vi "Read Source.vi"(8 "Error In":errorcluster, 11 "Node In":refnum<class "NonTerminal.lvclass">) -> (0 "Error Out":errorcluster, 2 "Source":string, 3 "Node Out":refnum<class "NonTerminal.lvclass">)   [LabVIEW 2018, in "Toolkit.lvlib" / "Nodes.lvlib" / "NonTerminal.lvclass"]
uses:
  NonTerminal.lvclass
  Abstract/Abstract.lvclass
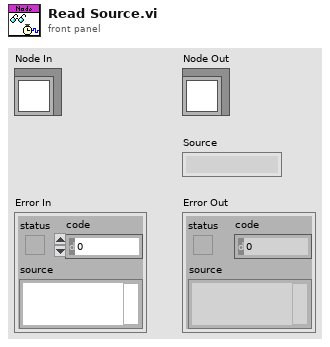
[diagram p1: front panel]
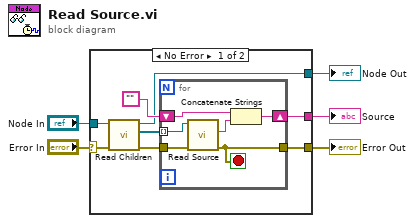
[diagram p0: block diagram]
diagram:
  n1 = case shown="No Error" "Error In" {
    selector: "Error In" -> [w10 w20]
    tunnel: "Node In" -> [w9 w21]
    tunnel: [w8 w21] -> w3
    tunnel: [w7 _] -> w2
    tunnel: [w6 w20] -> w1
    frame No Error {
      n2 = call-dynamic "Read Children.vi"("Error In"=w10, "Non-Terminal In"=w9) -> ("Error Out"=w11:errorcluster, "Children"=w12:refnum<class "Abstract.lvclass">[], "Non-Terminal Out"=w8:refnum<class "NonTerminal.lvclass">)  [unwired: 7 in]
      n3 = for {
        shift-right: [w18] -> w7
        shift-left: "" -> [w19]
        tunnel: w12 -> [w16] mode=indexing
        tunnel: w11 -> [w15]
        tunnel: [w14] -> w6
        stop <- w14 stop-if-true
        n4 = call-dynamic "Read Source.vi"("Error In"=w15, "Node In"=w16) -> ("Error Out"=w14:errorcluster, "Source"=w17:string)  [unwired: 7 in, 1 out]
        n5 = Concatenate Strings(w19, w17) -> (w18:string)
      }
    }
    frame Error {
    }
  }
  "Error Out" <- w1
  "Node Out" <- w3
  "Source" <- w2
